vi "Set getCANDatafromrgrpcServer_getFrameResponse.vi"(7 "Complete Call (T)":bool=TRUE, 8 "error in (no error)":errorcluster, 10 "Message Data":T1, 11 "gRPCid":T2) -> (0 "error out":errorcluster)   [LabVIEW 2020, in "server1.lvlib" / "server1.lvclass"]
uses:
  server1.lvclass
  gRPC lvSupport/Server API/typeDefs/grpcId.ctl
  dcc74a39-081a-4bdd-860b-8ed792803c96.vi
  gRPC lvSupport/Server API/Server/Get Server DLL Path.vi
  <vilib>/Utility/error.llb/Error Cluster From Error Code.vi
  server1.lvclass/server1.ctl
  gRPC lvSupport/gprc-lvsupport.lvlib
  getCANDatafromrgrpcServer_getFrameResponse_Data.ctl
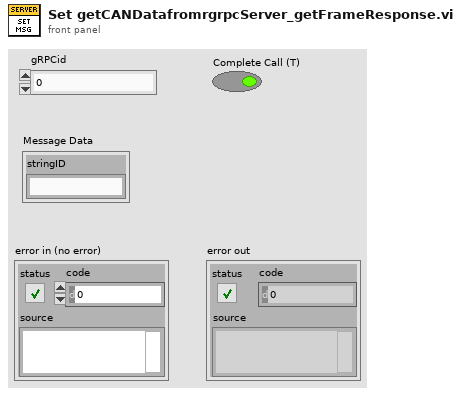
[diagram p1: front panel]
types:
  T1 = typedef "server1.lvlib/server1.lvclass/getCANDatafromrgrpcServer_getFrameResponse_Data.ctl" = cluster{"stringID":string}
  T2 = typedef "server1.lvlib/gprc-lvsupport.lvlib/grpcId.ctl" = u64
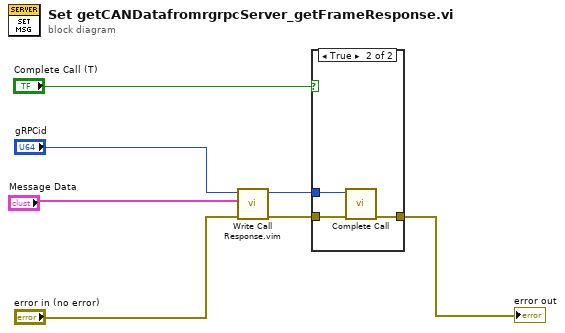
[diagram p0: block diagram]
diagram:
  n1 = call "Write Call Response.vim"("error in (no error)"="error in (no error)", "Response Data"="Message Data", "gRPCid in"="gRPCid") -> ("error out"=w4:errorcluster, "gRPCid"=w5:T2)  [unwired: 7 in]
  n2 = case shown="True" "Complete Call (T)" {
    tunnel: [w8 w11] -> w7
    tunnel: w5 -> [_ w10]
    tunnel: w4 -> [w8 w9]
    frame False {
    }
    frame True {
      n3 = call "Complete Call.vi"("gRPCid"=w10, "error in (no error)"=w9) -> ("error out"=w11:errorcluster)  [unwired: 8 in]
    }
  }
  "error out" <- w7
